vi "set ALS method.vi"(6 "Reagent volume (ul)":dbl[](array[numeric])=[5.0, 15.0], 7 "Reagent location":dbl[](array[numeric])=[1.0, 2.0], 9 "Mix vial Location":dbl=5.0, 10 "Wash vial Location":dbl=4.0, 11 "method folder":path=path "C:/Chem32 (new)/2/Methods/DropletSys.M") -> ()   [LabVIEW 2017]
panel:
  out "appended path":path
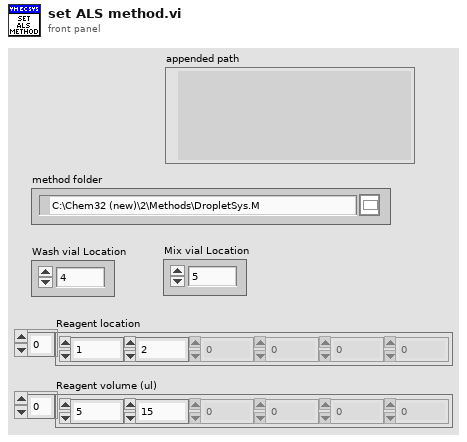
[diagram p1: front panel]
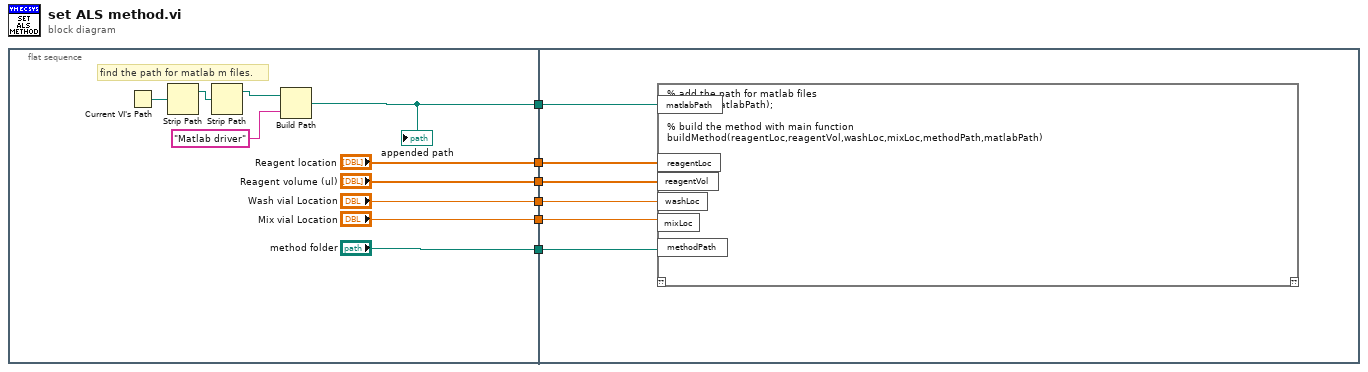
[diagram p0: block diagram]
diagram:
  n1 = flat-sequence {
    tunnel: [w12] -> w6
    tunnel: ["Wash vial Location"] -> w5
    tunnel: ["Mix vial Location"] -> w4
    tunnel: ["Reagent volume (ul)"] -> w3
    tunnel: ["Reagent location"] -> w2
    tunnel: ["method folder"] -> w1
    tunnel: w6 -> [w22]
    tunnel: w5 -> [w21]
    tunnel: w4 -> [w20]
    tunnel: w3 -> [w19]
    tunnel: w2 -> [w18]
    tunnel: w1 -> [w17]
    frame #0 {
      # "find the path for matlab m files."
      n2 = Current VI's Path() -> (path=w16:path)
      n3 = Strip Path(path=w16) -> (stripped path=w15:path)  [unwired: 1 out]
      n4 = Strip Path(path=w15) -> (stripped path=w14:path)  [unwired: 1 out]
      n5 = Build Path(base path=w14, name or relative path="Matlab driver") -> (appended path=w12:path)
      "appended path" <- w12
    }
    frame #1 {
      n6 = script code="% add the path for matlab files\naddpath(matlabPath);\n\n% build the method with main function\nbuildMethod(reagentLoc,reagentVol,washLoc,mixLoc,methodPath,matlabPath)"("matlabPath"=w22, "reagentLoc"=w18, "reagentVol"=w19, "washLoc"=w21, "mixLoc"=w20, "methodPath"=w17) -> ()  [unwired: 1 in, 1 out]
    }
  }
